vi "WS1050 Bench CAP Characterization_Ver1.2.vi"() -> ()   [LabVIEW 2012]
panel:
  in  "Tab Control":enum32{"CONTROL", "INDICATION"}(tab)
  in  "RFFE Com Port":refnum<visa-resource-name>="COM3"
  in  "AD7747 Com Port":refnum<visa-resource-name>="COM1"
  in  "Init":bool=TRUE
  in  "Wafer":string="WS1050"
  in  "Lot":string="Toggle 7"
  in  "SN":string="01"
  in  "Temperature":string="RT"
  in  "Delay(ms)":u32=100
  in  "TMN DC\\CAP Data Log File Path":path=path "C:/Andy Tr/Temp"
  in  "String":string="WS1050 BENCH CAP CHARACTERIZATION Ver1.2"
  out "C3Cal (pF)":dbl=-4.9974111328125
  out "C1Cal (pF)":dbl=-4.5642919921875
  out "C2Cal (pF)":dbl=-4.9191376953125
  out "S_ValueC3(pF)":dbl=-4.9974111328125
  out "S_ValueC1(pF)":dbl=-4.5642919921875
  out "S_ValueC2(pF)":dbl=-4.9191376953125
  in  "Calib Socket":bool
  out "C1_Mesa(pF)":dbl
  out "C2_Mesa(pF)":dbl
  out "C3_Mesa(pF)":dbl
  in  "A364X_VDD":refnum<visa-resource-name>="GPIB1::6::INSTR"
  in  "IDD Limit":dbl=0.02 format="%.2p"
  in  "VDD":dbl=3.3
  in  "CP Setting":i32(ring) items=["CP OFF", "CP ON", "DVA OFF", "DVA ON", "ECAL OFF", "ECAL ON", "CP 40.25V", "CP 35V", "CP 38V", "CP 44V", "CP 50V", "CP 23.75V", "CP 25.25V", "CP 29.75V", "C1 ON", "C1 OFF", "C2 ON", "C2 OFF", "C3 ON", "C3 OFF"]
  in  "Send":bool
  in  "Init AD7747":bool
  in  "Keithley 2000":refnum<visa-resource-name>
  in  "CApDac_values":string[](array[string])=["900b99", "900b99", "900b9b"]
  in  "Toggle Relay":bool
  in  "A3631E":refnum<visa-resource-name>
  in  "Channel":i32(ring)=1 items=["Channel 1"=1, "Channel 2"=2, "Channel 3"=3]
  in  "Relay Delay (s)":u32
  out "C_min(pF)":string[](array[string])
  out "C_Max":string[](array[string])
  out "C_Min2(pF)":string[](array[string])
  out "error out":errorcluster
  in  "error in (no error)":errorcluster
  in  "stop":bool
  in  "Abort":bool
  in  "Start Test":bool
  out "Running loop":i32
  in  "Set Cmax":string[](array[string])=["07413B", "07423B", "07433B"]
  out "Status":string="Relays Open..."
  # "This Version is working with V1.9 Marketing Firmware"
  # "Company:  WiSpry Inc\n198 Fairbanks Ste 198 Irvine\n\nCreated by:  Andy V Tran\nDate:  03/11/2015\nTP:  WS1050 Bench\nCAP Characterization"
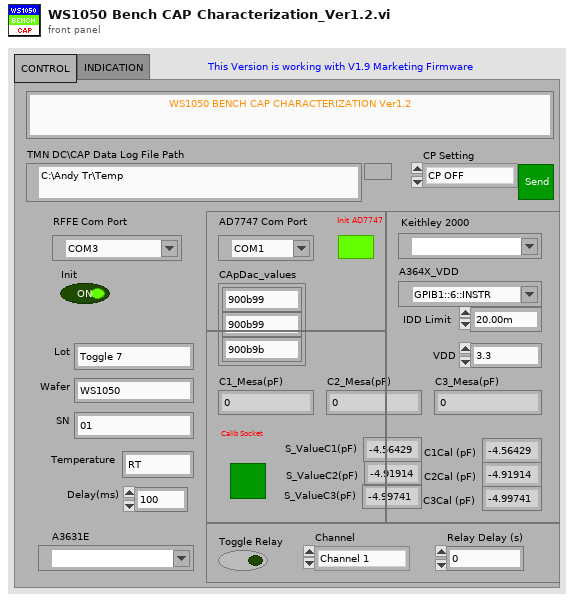
[diagram p1: front panel]
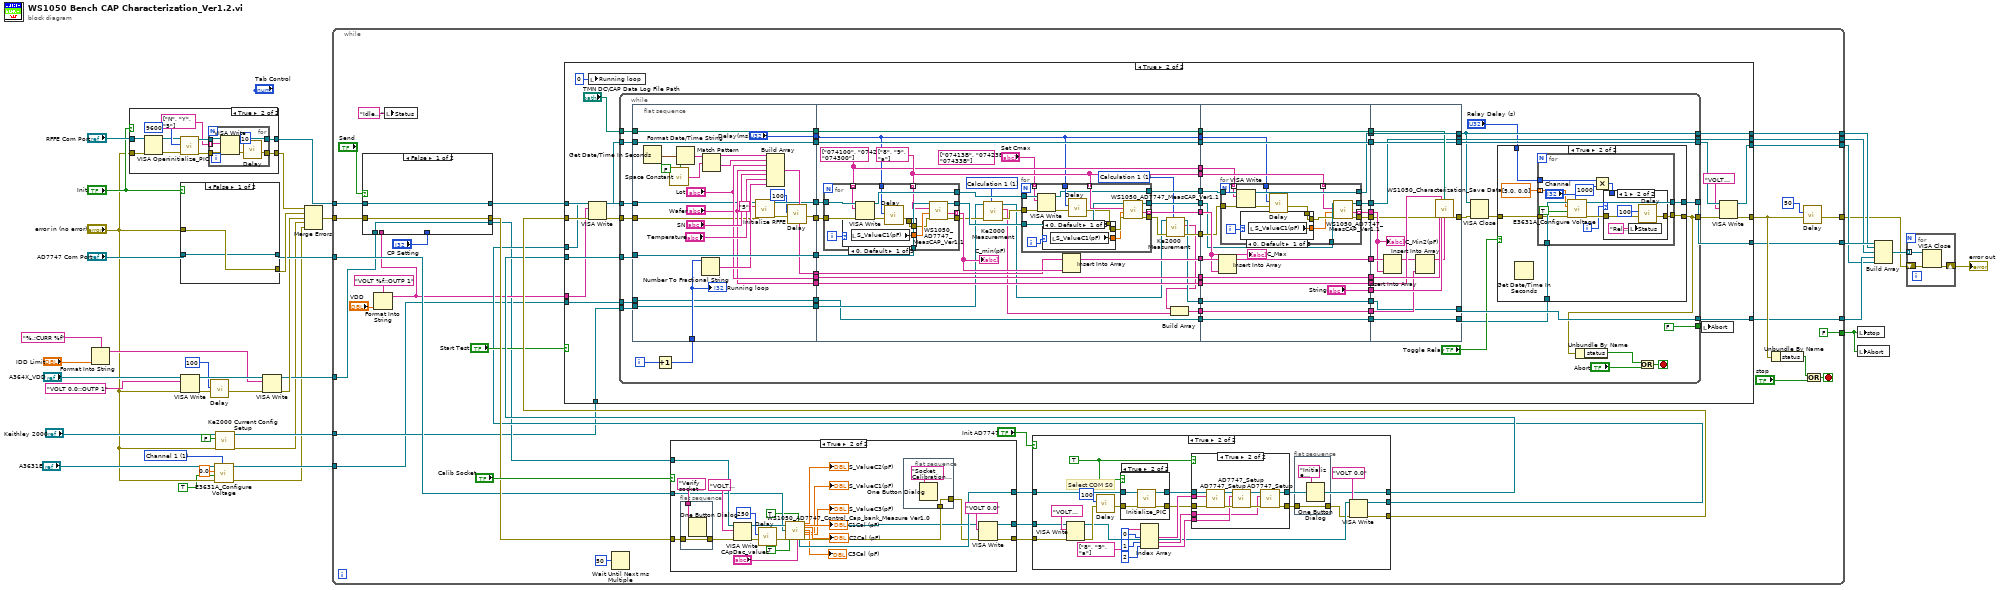
[diagram p0: block diagram]
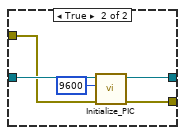
[diagram p3: hidden frame]
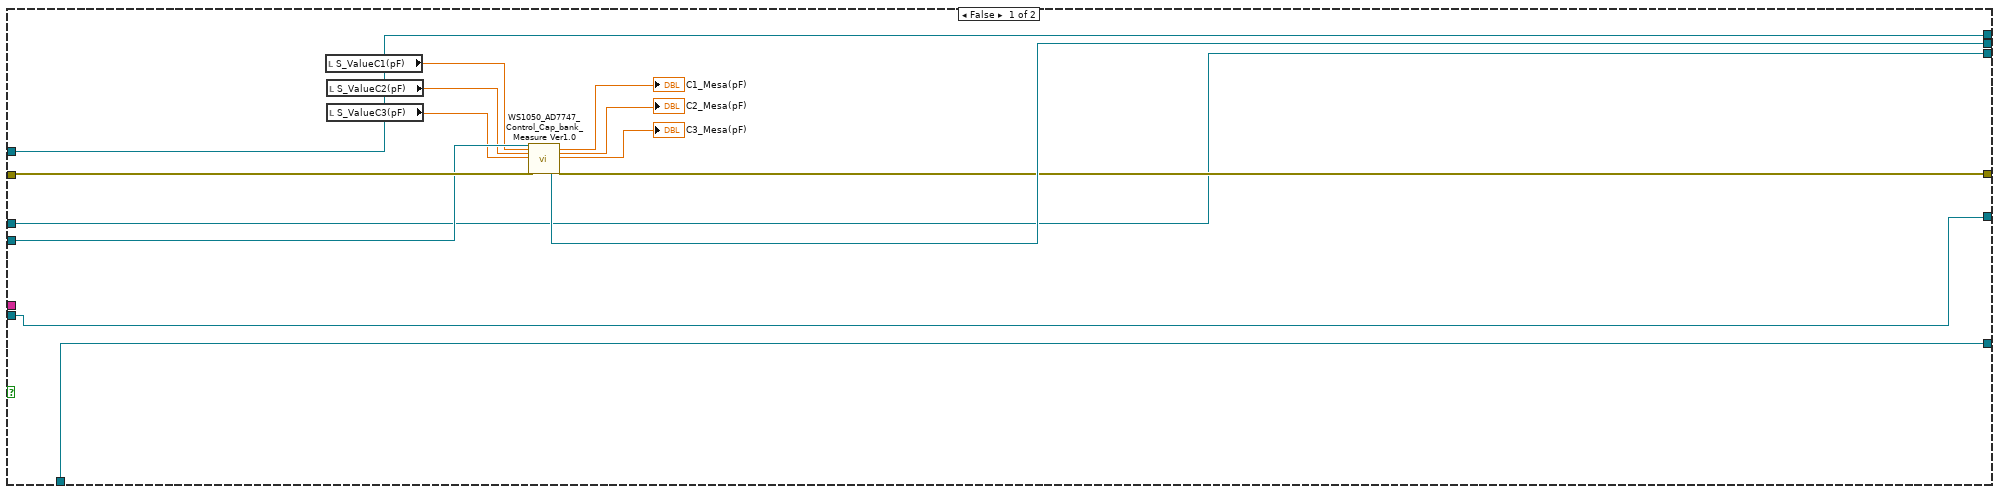
[diagram p8: hidden frame]
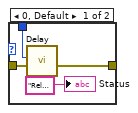
[diagram p10: hidden frame]
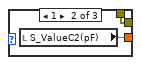
[diagram p11: hidden frame]
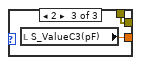
[diagram p12: hidden frame]
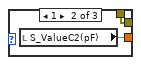
[diagram p13: hidden frame]
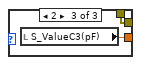
[diagram p14: hidden frame]
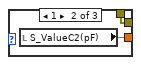
[diagram p15: hidden frame]
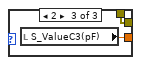
[diagram p16: hidden frame]
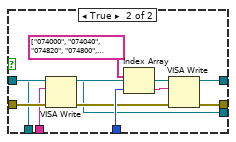
[diagram p17: hidden frame]
diagram:
  w13 = 1 items=["Channel 1"=1, "Channel 2"=2, "Channel 3"=3] ("Channel (1: Channel 1)")
  n1 = Format Into String(format string="%.;CURR %f", "IDD Limit") -> (resulting string=w34:string)  [unwired: 2 in, 1 out]
  n2 = case shown="True" "Init" {
    tunnel: "error in (no error)" -> [w41 w46]
    tunnel: [w41 w51] -> w17
    tunnel: "RFFE Com Port" -> [w40 w43]
    tunnel: [w40 w50] -> w18
    frame False {
    }
    frame True {
      n3 = VISA Open(error in (no error)=w46, VISA resource name=w43) -> (VISA resource name=w44:refnum<visa-resource-name>, error out=w45:errorcluster)  [unwired: 3 in]
      n4 = call "initialize_PIC.vi"("error in (no error)"=w45, "baud rate"=u32 9600, "Select Com Port"=w44) -> ("error out"=w48:errorcluster, "VISA resource name out"=w49:refnum<visa-resource-name>)  [unwired: 7 in]
      n5 = for {
        tunnel: [w58] -> w51
        tunnel: [w52] -> w50
        tunnel: w49 -> [w53]
        tunnel: w48 -> [w55]
        tunnel: string[] ["N", "Y", "5"] -> [w54] mode=indexing
        n6 = VISA Write(VISA resource name=w53, write buffer=w54, error in (no error)=w55) -> (VISA resource name out=w52:refnum<visa-resource-name>, error out=w56:errorcluster)  [unwired: 1 out]
        n7 = call "Delay.vi"("error in (no error)"=w56, "milliseconds to wait"=u32 10) -> ("error out"=w58:errorcluster)  [unwired: 9 in]
      }
    }
  }
  n8 = case shown="False" "Init" {
    tunnel: "AD7747 Com Port" -> [w59 w64]
    tunnel: [w60 w63] -> w38
    tunnel: [w59 w62] -> w37
    tunnel: "error in (no error)" -> [w60 w61]
    frame False {
    }
    frame True {
      n9 = call "Initialize_PIC.vi"("error in (no error)"=w61, "baud rate"=u32 9600, "Select Com Port"=w64) -> ("error out"=w63:errorcluster, "VISA resource name out"=w62:refnum<visa-resource-name>)  [unwired: 7 in]
    }
  }
  n10 = VISA Write(VISA resource name="A364X_VDD", write buffer="VOLT 0.0;:OUTP 1", error in (no error)="error in (no error)") -> (VISA resource name out=w35:refnum<visa-resource-name>, error out=w31:errorcluster)  [unwired: 1 out]
  n11 = call "Delay.vi"("error in (no error)"=w31, "milliseconds to wait"=u32 100) -> ("error out"=w36:errorcluster)  [unwired: 9 in]
  n12 = call "E3631A_Configure Voltage.vi"("Channel (1: Channel 1)"=w13, "error in (no error)"="error in (no error)", "Enable Output (T: Enable)"=TRUE, "Voltage(V)"=0.0, "VISA resource name"="A3631E") -> ("error out"=w10:errorcluster, "VISA resource name 2"=w11:refnum<visa-resource-name>)  [unwired: 5 in]
  n13 = call "Ke2000 Current Config Setup.vi"("error in (no error)"="error in (no error)", "Auto Range(T/F)"=FALSE, "VISA resource name"="Keithley 2000") -> ("error out"=w21:errorcluster, "VISA resource name out"=w22:refnum<visa-resource-name>)  [unwired: 7 in]
  n14 = VISA Write(VISA resource name=w35, write buffer=w34, error in (no error)=w36) -> (VISA resource name out=w26:refnum<visa-resource-name>, error out=w27:errorcluster)  [unwired: 1 out]
  n15 = Merge Errors(w17, w38, w27, w21, w10) -> (w9:errorcluster)
  n16 = while {
    tunnel: w18 -> [w99]
    tunnel: w9 -> [w100]
    tunnel: w37 -> [w87]
    tunnel: [w95] -> w2
    tunnel: [w93] -> w7
    tunnel: [w92] -> w6
    tunnel: w26 -> [w74]
    tunnel: [w78] -> w4
    tunnel: [FALSE ("stop")] -> w25
    tunnel: w22 -> [w70]
    tunnel: [w69] -> w5
    tunnel: w11 -> [w68]
    tunnel: [w67] -> w8
    stop <- w90 stop-if-true
    n17 = Format Into String(format string="VOLT %f;:OUTP 1", "VDD") -> (resulting string=w73:string)  [unwired: 2 in, 1 out]
    n18 = case shown="False" "Send" {
      tunnel: w100 -> [w469 w475]
      tunnel: [w469 w479] -> w88
      tunnel: [w468 w478] -> w98
      tunnel: "CP Setting" -> [_ w477]
      tunnel: w99 -> [w468 w476]
      tunnel: w74 -> [w467 w474]
      tunnel: w73 -> [_ w473]
      tunnel: [w467 w471] -> w72
      frame False {
      }
      frame True {
        n19 = VISA Write(VISA resource name=w474, write buffer=w473, error in (no error)=w475) -> (VISA resource name out=w471:refnum<visa-resource-name>, error out=w472:errorcluster)  [unwired: 1 out]
        n20 = Index Array(array=string[] ["074000", "074040", "074820", "074800", "074044", "074040", "074776", "07476F", "074773", "07477B", "07477C", "074760", "074762", "074768", "07413B", "074100", "07423B", "074200", "07433B", "074300"], index=w477) -> (element=w480:string)
        n21 = VISA Write(VISA resource name=w476, write buffer=w480, error in (no error)=w472) -> (VISA resource name out=w478:refnum<visa-resource-name>, error out=w479:errorcluster)  [unwired: 1 out]
      }
    }
    n22 = local write "Status"("Idle..." ("Status")) -> ()
    n23 = Wait Until Next ms Multiple(millisecond multiple=u32 50) -> ()  [unwired: 1 out]
    n24 = case shown="True" "Calib Socket" {
      tunnel: w88 -> [w153 w177]
      tunnel: [w153 w160] -> w82
      tunnel: w87 -> [w152 w158]
      tunnel: w72 -> [w151 w166]
      tunnel: [w151 w161] -> w83
      tunnel: [w152 w175] -> w81
      frame False {
      }
      frame True {
        n25 = flat-sequence {
          tunnel: [w180] -> w167
          tunnel: w177 -> [w180]
          tunnel: "Verify socket should be empty" ("message") -> [w179]
          frame #0 {
            n26 = One Button Dialog(message=w179) -> ()  [unwired: 1 in, 1 out]
          }
        }
        n27 = VISA Write(VISA resource name=w166, write buffer="VOLT 3.3;:OUTP 1", error in (no error)=w167) -> (VISA resource name out=w162:refnum<visa-resource-name>, error out=w164:errorcluster)  [unwired: 1 out]
        n28 = call "Delay.vi"("error in (no error)"=w164, "milliseconds to wait"=u32 250) -> ("error out"=w157:errorcluster)  [unwired: 9 in]
        n29 = call "WS1050_AD7747_Control_Cap_bank_Measure Ver1.0.vi"("Select Com Port"=w158, "errorin"=w157, "Push Button to Measue Cap"=TRUE, "CApDac_values"="CApDac_values", "Push Button to Calibrate"=TRUE ("Push Button to Initialize AD7747")) -> ("Com Port Out"=w175:refnum<visa-resource-name>, "C2(pF)"=→"S_ValueC2(pF)":dbl, "C1_Mesa(pF)"=→"C1Cal (pF)":dbl, "C2_Mesa(pF)"=→"C2Cal (pF)":dbl, "C3_Mesa(pF)"=→"C3Cal (pF)":dbl, "C1(pF)"=→"S_ValueC1(pF)":dbl, "C3(pF)"=→"S_ValueC3(pF)":dbl, "error out"=w176:errorcluster)  [unwired: 15 in]
        n30 = flat-sequence {
          tunnel: [w181] -> w159
          tunnel: w176 -> [w181]
          frame #0 {
            n31 = One Button Dialog(message="Socket Calibration Completed, Please insert DUT into the Socket") -> ()  [unwired: 1 in, 1 out]
          }
        }
        n32 = VISA Write(VISA resource name=w162, write buffer="VOLT 0.0", error in (no error)=w159) -> (VISA resource name out=w161:refnum<visa-resource-name>, error out=w160:errorcluster)  [unwired: 1 out]
      }
    }
    n33 = case shown="True" "Init AD7747" {
      tunnel: w81 -> [w104 w129]
      tunnel: [w105 w109] -> w85
      tunnel: w82 -> [w105 w114]
      tunnel: [w104 w107] -> w84
      tunnel: w83 -> [w103 w115]
      tunnel: [w103 w110] -> w79
      frame False {
      }
      frame True {
        w119 = TRUE
        # "Select COM S0"
        n34 = VISA Write(VISA resource name=w115, write buffer="VOLT 3.3;:OUTP 1", error in (no error)=w114) -> (VISA resource name out=w111:refnum<visa-resource-name>, error out=w113:errorcluster)  [unwired: 1 out]
        n35 = call "Delay.vi"("error in (no error)"=w113, "milliseconds to wait"=u32 100) -> ("error out"=w117:errorcluster)  [unwired: 9 in]
        n36 = case shown="True" w119 {
          tunnel: [w143 w148] -> w120
          tunnel: [w144 w147] -> w128
          tunnel: w129 -> [w144 w146]
          tunnel: w117 -> [w143 w145]
          frame False {
          }
          frame True {
            n37 = call "Initialize_PIC.vi"("error in (no error)"=w145, "Select Com Port"=w146) -> ("error out"=w148:errorcluster, "VISA resource name out"=w147:refnum<visa-resource-name>)  [unwired: 8 in]
          }
        }
        n38 = Index Array(array=string[] ["8", "9", "a"], index #1=0 ("index"), index #2=1 ("index"), index #3=2 ("index")) -> (element #1=w123:string, element #2=w122:string, element #3=w121:string)
        n39 = case shown="True" w119 {
          tunnel: w120 -> [w131 w134]
          tunnel: [w131 w132] -> w106
          tunnel: w128 -> [w130 w142]
          tunnel: w123 -> [_ w137]
          tunnel: w121 -> [_ w136]
          tunnel: w122 -> [_ w135]
          tunnel: [w130 w133] -> w107
          frame False {
          }
          frame True {
            n40 = call "AD7747_Setup.vi"("error in"=w134, "AD7747_Number"=w137, "Control"=w142) -> ("error out"=w141:errorcluster, "Control out"=w140:refnum<visa-resource-name>)  [unwired: 6 in, 1 out]
            n41 = call "AD7747_Setup.vi"("error in"=w141, "AD7747_Number"=w136, "Control"=w140) -> ("error out"=w139:errorcluster, "Control out"=w138:refnum<visa-resource-name>)  [unwired: 6 in, 1 out]
            n42 = call "AD7747_Setup.vi"("error in"=w139, "AD7747_Number"=w135, "Control"=w138) -> ("error out"=w132:errorcluster, "Control out"=w133:refnum<visa-resource-name>)  [unwired: 6 in, 1 out]
          }
        }
        n43 = flat-sequence {
          tunnel: w106 -> [w149]
          tunnel: [w149] -> w108
          frame #0 {
            n44 = One Button Dialog(message="Initialize AD7747 completed!") -> ()  [unwired: 1 in, 1 out]
          }
        }
        n45 = VISA Write(VISA resource name=w111, write buffer="VOLT 0.0", error in (no error)=w108) -> (VISA resource name out=w110:refnum<visa-resource-name>, error out=w109:errorcluster)  [unwired: 1 out]
      }
    }
    n46 = case shown="True" "Start Test" {
      tunnel: w98 -> [w189 w217]
      tunnel: w85 -> [w196 w212]
      tunnel: w84 -> [w195 w216]
      tunnel: [w193 w210] -> w96
      tunnel: [w189 w215] -> w93
      tunnel: [w194 w214] -> w92
      tunnel: w79 -> [w188 w211]
      tunnel: [w188 w207] -> w78
      tunnel: w73 -> [_ w202]
      tunnel: w70 -> [w184 w200]
      tunnel: [w184 w199] -> w69
      tunnel: w68 -> [w183 w198]
      tunnel: [w183 w197] -> w67
      frame False {
        n47 = local read "S_ValueC1(pF)"() -> (w187:dbl)
        n48 = local read "S_ValueC2(pF)"() -> (w186:dbl)
        n49 = local read "S_ValueC3(pF)"() -> (w185:dbl)
        n50 = call "WS1050_AD7747_Control_Cap_bank_Measure Ver1.0.vi"("Select Com Port"=w195, "S_Value C1"=w187, "S_Value C2"=w186, "S_Value C3"=w185, "errorin"=w196) -> ("Com Port Out"=w194:refnum<visa-resource-name>, "C1_Mesa(pF)"=→"C1_Mesa(pF)":dbl, "C2_Mesa(pF)"=→"C2_Mesa(pF)":dbl, "C3_Mesa(pF)"=→"C3_Mesa(pF)":dbl, "error out"=w193:errorcluster)  [unwired: 15 in, 3 out]
      }
      frame True {
        n51 = VISA Write(VISA resource name=w211, write buffer=w202, error in (no error)=w212) -> (VISA resource name out=w209:refnum<visa-resource-name>, error out=w213:errorcluster)  [unwired: 1 out]
        n52 = local write "Running loop"(0 ("Loop Running")) -> ()
        n53 = while {
          tunnel: w217 -> [w277]
          tunnel: w213 -> [w276]
          tunnel: w216 -> [w275]
          tunnel: [w218] -> w206
          tunnel: "TMN DC\\CAP Data Log File Path" -> [w270]
          tunnel: [w236] -> w215
          tunnel: [w266] -> w214
          tunnel: w209 -> [w262]
          tunnel: [w259] -> w208
          tunnel: [FALSE ("Abort")] -> w203
          tunnel: w200 -> [w234]
          tunnel: [w228] -> w199
          tunnel: w198 -> [w225]
          tunnel: [w220] -> w197
          i -> [w253]
          stop <- w272 stop-if-true
          n54 = flat-sequence {
            tunnel: w262 -> [w332]
            tunnel: w270 -> [w333]
            tunnel: w275 -> [w334]
            tunnel: w276 -> [w315]
            tunnel: w277 -> [w316]
            tunnel: [w312] -> w251
            tunnel: [w313] -> w250
            tunnel: [w334] -> w249
            tunnel: [w333] -> w248
            tunnel: [w332] -> w247
            tunnel: w246 -> [w319]
            tunnel: [w322] -> w245
            tunnel: ["Lot"] -> w244
            tunnel: ["Wafer"] -> w241
            tunnel: ["Delay(ms)"] -> w237
            tunnel: w234 -> [w310]
            tunnel: [w310] -> w233
            tunnel: w225 -> [w309]
            tunnel: [w309] -> w224
            tunnel: [w356] -> w280
            tunnel: [w361] -> w279
            tunnel: [w343] -> w274
            tunnel: [w360] -> w269
            tunnel: [w359] -> w267
            tunnel: [w358] -> w264
            tunnel: [w355] -> w260
            tunnel: [w354] -> w258
            tunnel: [w349] -> w257
            tunnel: [w353] -> w256
            tunnel: w251 -> [w366]
            tunnel: w250 -> [w365]
            tunnel: w249 -> [w363]
            tunnel: w248 -> [w358]
            tunnel: w247 -> [w355]
            tunnel: w245 -> [w352]
            tunnel: w244 -> [w351]
            tunnel: [w351] -> w243
            tunnel: w241 -> [w350]
            tunnel: [w350] -> w240
            tunnel: w237 -> [w349]
            tunnel: w233 -> [w346]
            tunnel: [w341] -> w232
            tunnel: [w337] -> w230
            tunnel: w224 -> [w335]
            tunnel: [w335] -> w223
            tunnel: w280 -> [w429]
            tunnel: w279 -> [w428]
            tunnel: [w427] -> w278
            tunnel: w274 -> [w423]
            tunnel: [w424] -> w273
            tunnel: w269 -> [w419]
            tunnel: [w418] -> w268
            tunnel: w267 -> [w417]
            tunnel: [w426] -> w265
            tunnel: w264 -> [w426]
            tunnel: [w425] -> w261
            tunnel: w260 -> [w425]
            tunnel: w258 -> [w422]
            tunnel: w257 -> [w421]
            tunnel: w256 -> [w420]
            tunnel: [w416] -> w255
            tunnel: [w415] -> w254
            tunnel: w243 -> [w414]
            tunnel: [w414] -> w242
            tunnel: w240 -> [w413]
            tunnel: [w413] -> w239
            tunnel: ["String"] -> w238
            tunnel: w232 -> [w411]
            tunnel: [w411] -> w231
            tunnel: w230 -> [w410]
            tunnel: [w410] -> w229
            tunnel: w223 -> [w409]
            tunnel: [w409] -> w222
            tunnel: w278 -> [w461]
            tunnel: w273 -> [w456]
            tunnel: [w466] -> w235
            tunnel: w268 -> [w465]
            tunnel: [w465] -> w236
            tunnel: [w462] -> w266
            tunnel: w265 -> [w464]
            tunnel: w261 -> [w463]
            tunnel: [w463] -> w259
            tunnel: w255 -> [w462]
            tunnel: w254 -> [w460]
            tunnel: w242 -> [w459]
            tunnel: w239 -> [w458]
            tunnel: w238 -> [w457]
            tunnel: w231 -> [w452]
            tunnel: w229 -> [w454]
            tunnel: [w452] -> w228
            tunnel: w222 -> [w451]
            tunnel: [w451] -> w221
            frame #0 {
              n55 = Get Date/Time In Seconds() -> (seconds since 1Jan1904=w328:timestamp)
              n56 = call <vilib>:"Space Constant.vi"() -> ("String"=w331:string)
              n57 = Format Date/Time String(seconds (now)=w328, UTC format=FALSE) -> (date/time string=w329:string)  [unwired: 1 out]
              n58 = Number To Fractional String(number=w319) -> (F-format string=w323:string)  [unwired: 3 in]
              n59 = Match Pattern(string=w329, regular expression=w331) -> (before substring=w327:string, after substring=w326:string)  [unwired: 3 out]
              n60 = call "Initialize RFFE.vi"("error in (no error)"=w315, "write buffer"="5", "Select Com Port"=w316) -> ("error out"=w314:errorcluster, "VISA resource name out"=w312:refnum<visa-resource-name>)  [unwired: 7 in]
              n61 = Build Array(w327, w326, "Lot", "Wafer", "SN", "Temperature", w323) -> (w322:string[])
              n62 = call "Delay.vi"("error in (no error)"=w314, "milliseconds to wait"=u32 100) -> ("error out"=w313:errorcluster)  [unwired: 9 in]
              "Running loop" <- w319
            }
            frame #1 {
              w340 = u16 1 items=["Function", "Calculation 1", "Calculation 2", "Calculation 3"] ("Source (0: Function)")
              w345 = u16 1 items=["Function", "Calculation 1", "Calculation 2", "Calculation 3"] ("Source (0: Function)")
              w354 = string[] ["8", "9", "a"]
              (unwired) string[] ["07413B", "07423B", "07433B"]
              w353 = string[] ["074100", "074200", "074300"]
              n63 = for {
                tunnel: w366 -> [w402]
                tunnel: w365 -> [w401]
                tunnel: w353 -> [w400] mode=indexing
                tunnel: [w399] -> w364
                tunnel: w363 -> [w398]
                tunnel: [w397] -> w362
                tunnel: [w396] -> w347
                tunnel: w349 -> [w394]
                tunnel: w354 -> [w393] mode=indexing
                tunnel: [w392] -> w357 mode=indexing
                i -> [w391]
                n64 = VISA Write(VISA resource name=w402, write buffer=w400, error in (no error)=w401) -> (VISA resource name out=w399:refnum<visa-resource-name>, error out=w395:errorcluster)  [unwired: 1 out]
                n65 = call "Delay.vi"("error in (no error)"=w395, "milliseconds to wait"=w394) -> ("error out"=w389:errorcluster)  [unwired: 9 in]
                n66 = case shown="0, Default" w391 {
                  tunnel: [w404 w406 w408] -> w390
                  tunnel: w389 -> [w403 w405 w407]
                  tunnel: [w403 w405 w407] -> w388
                  frame 0, Default {
                    n67 = local read "S_ValueC1(pF)"() -> (w404:dbl)
                  }
                  frame 1 {
                    n68 = local read "S_ValueC2(pF)"() -> (w406:dbl)
                  }
                  frame 2 {
                    n69 = local read "S_ValueC3(pF)"() -> (w408:dbl)
                  }
                }
                n70 = call "WS1050_AD7747_MeasCAP_Ver1.1.vi"("error in (no error)"=w388, "OFFSet Cal"=w390, "AD7747_Number"=w393, "Control"=w398) -> ("error"=w396:errorcluster, "CAP (pF)"=w392:string, "Control out"=w397:refnum<visa-resource-name>)  [unwired: 3 in, 2 out]
              }
              "C_min(pF)" <- w357
              n71 = call "Ke2000 Measurement.vi"("Source (0: Function)"=w345, "error in (no error)"=w347, "VISA resource name"=w346) -> ("error out"=w348:errorcluster, "Meas in micro"=w338:string, "VISA resource name out"=w342:refnum<visa-resource-name>)  [unwired: 3 in, 3 out]
              n72 = for {
                tunnel: w364 -> [w381]
                tunnel: w348 -> [w380]
                tunnel: "Set Cmax" -> [w379] mode=indexing
                tunnel: w349 -> [w377]
                tunnel: w354 -> [w376] mode=indexing
                tunnel: [w375] -> w344
                tunnel: [w374] -> w359
                tunnel: [w373] -> w360
                tunnel: w362 -> [w372]
                tunnel: [w371] -> w361 mode=indexing
                i -> [w369]
                n73 = VISA Write(VISA resource name=w381, write buffer=w379, error in (no error)=w380) -> (VISA resource name out=w373:refnum<visa-resource-name>, error out=w378:errorcluster)  [unwired: 1 out]
                n74 = call "Delay.vi"("error in (no error)"=w378, "milliseconds to wait"=w377) -> ("error out"=w368:errorcluster)  [unwired: 9 in]
                n75 = case shown="0, Default" w369 {
                  tunnel: [w383 w385 w387] -> w367
                  tunnel: w368 -> [w382 w384 w386]
                  tunnel: [w382 w384 w386] -> w370
                  frame 0, Default {
                    n76 = local read "S_ValueC1(pF)"() -> (w383:dbl)
                  }
                  frame 1 {
                    n77 = local read "S_ValueC2(pF)"() -> (w385:dbl)
                  }
                  frame 2 {
                    n78 = local read "S_ValueC3(pF)"() -> (w387:dbl)
                  }
                }
                n79 = call "WS1050_AD7747_MeasCAP_Ver1.1.vi"("error in (no error)"=w370, "OFFSet Cal"=w367, "AD7747_Number"=w376, "Control"=w372) -> ("error"=w375:errorcluster, "CAP (pF)"=w371:string, "Control out"=w374:refnum<visa-resource-name>)  [unwired: 3 in, 2 out]
              }
              n80 = Insert Into Array(array=w352, new element=w357) -> (w356:string[])  [unwired: 1 in]
              n81 = call "Ke2000 Measurement.vi"("Source (0: Function)"=w340, "error in (no error)"=w344, "VISA resource name"=w342) -> ("error out"=w343:errorcluster, "Meas in micro"=w339:string, "VISA resource name out"=w341:refnum<visa-resource-name>)  [unwired: 3 in, 3 out]
              n82 = Build Array(w339, w338) -> (w337:string[])
            }
            frame #2 {
              n83 = Insert Into Array(array=w429, new element=w428) -> (w427:string[])  [unwired: 1 in]
              n84 = for {
                tunnel: w419 -> [w444]
                tunnel: w423 -> [w443]
                tunnel: w420 -> [w442] mode=indexing
                tunnel: [w441] -> w418
                tunnel: w417 -> [w440]
                tunnel: [w439] -> w416
                tunnel: [w438] -> w424
                tunnel: w421 -> [w436]
                tunnel: w422 -> [w435] mode=indexing
                tunnel: [w434] -> w415 mode=indexing
                i -> [w433]
                n85 = VISA Write(VISA resource name=w444, write buffer=w442, error in (no error)=w443) -> (VISA resource name out=w441:refnum<visa-resource-name>, error out=w437:errorcluster)  [unwired: 1 out]
                n86 = call "Delay.vi"("error in (no error)"=w437, "milliseconds to wait"=w436) -> ("error out"=w431:errorcluster)  [unwired: 9 in]
                n87 = case shown="0, Default" w433 {
                  tunnel: [w446 w448 w450] -> w430
                  tunnel: w431 -> [w445 w447 w449]
                  tunnel: [w445 w447 w449] -> w432
                  frame 0, Default {
                    n88 = local read "S_ValueC1(pF)"() -> (w446:dbl)
                  }
                  frame 1 {
                    n89 = local read "S_ValueC2(pF)"() -> (w448:dbl)
                  }
                  frame 2 {
                    n90 = local read "S_ValueC3(pF)"() -> (w450:dbl)
                  }
                }
                n91 = call "WS1050_AD7747_MeasCAP_Ver1.1.vi"("error in (no error)"=w432, "OFFSet Cal"=w430, "AD7747_Number"=w435, "Control"=w440) -> ("error"=w438:errorcluster, "CAP (pF)"=w434:string, "Control out"=w439:refnum<visa-resource-name>)  [unwired: 3 in, 2 out]
              }
              "C_Max" <- w428
            }
            frame #3 {
              n92 = Insert Into Array(array=w461, new element=w460) -> (w455:string[])  [unwired: 1 in]
              n93 = Insert Into Array(array=w455, new element=w454) -> (w453:string[])  [unwired: 1 in]
              n94 = call "WS1050_Characterization_Save Data.vi"("error in (no error)"=w456, "Lot"=w459, "Wafer"=w458, "TP"=w457, "TMN DC\\CAP Data Log File Path"=w464, "All Out"=w453) -> ("error out"=w466:errorcluster)  [unwired: 19 in, 2 out]
              "C_Min2(pF)" <- w460
            }
          }
          n95 = Increment(x=w253) -> (x+1=w246:i32)
          n96 = VISA Close(VISA resource name=w236, error in (no error)=w235) -> (error out=w227:errorcluster)
          n97 = case shown="True" "Toggle Relay" {
            tunnel: w227 -> [w282 w288]
            tunnel: [w282 w287] -> w218
            tunnel: w221 -> [w281 w286]
            tunnel: [w281 w285] -> w220
            tunnel: "Relay Delay (s)" -> [_ w283]
            frame False {
            }
            frame True {
              n98 = Get Date/Time In Seconds() -> ()  [unwired: 1 out]
              n99 = for {
                tunnel: w288 -> [w297]
                tunnel: [w300] -> w287
                tunnel: w286 -> [w298]
                tunnel: [w295] -> w285
                tunnel: dbl[] [5.0, 0.0] -> [w293] mode=indexing
                tunnel: w283 -> [w292]
                i -> [w289]
                n100 = call "E3631A_Configure Voltage.vi"("Channel (1: Channel 1)"="Channel", "error in (no error)"=w297, "Enable Output (T: Enable)"=TRUE, "Voltage(V)"=w293, "VISA resource name"=w298) -> ("error out"=w299:errorcluster, "VISA resource name 2"=w295:refnum<visa-resource-name>)  [unwired: 5 in]
                n101 = Multiply(x=w292, y=u32 1000) -> (x*y=w290:u32)
                n102 = case shown="1" w289 {
                  tunnel: [w304 w308] -> w300
                  tunnel: w299 -> [w303 w307]
                  tunnel: w290 -> [w302 _]
                  frame 0, Default {
                    n103 = call "Delay.vi"("error in (no error)"=w303, "milliseconds to wait"=w302) -> ("error out"=w304:errorcluster)  [unwired: 9 in]
                    "Status" <- "Relays Open! Waiting for the next measurement..."
                  }
                  frame 1 {
                    n104 = local write "Status"("Relays Close! Measuring..." ("Status")) -> ()
                    n105 = call "Delay.vi"("error in (no error)"=w307, "milliseconds to wait"=u32 100) -> ("error out"=w308:errorcluster)  [unwired: 9 in]
                  }
                }
              }
            }
          }
          n106 = Unbundle By Name(w218) -> ("status"=w271:bool)
          n107 = Or(x=w271, y="Abort") -> (x .or. y?=w272:bool)
        }
        n108 = local write "Abort"(w203) -> ()
        n109 = VISA Write(VISA resource name=w208, write buffer="VOLT 0.0;:OUTP 0", error in (no error)=w206) -> (VISA resource name out=w207:refnum<visa-resource-name>, error out=w210:errorcluster)  [unwired: 1 out]
      }
    }
    n110 = Unbundle By Name(w96) -> ("status"=w97:bool)
    n111 = call "Delay.vi"("error in (no error)"=w96, "milliseconds to wait"=u32 50) -> ("error out"=w95:errorcluster)  [unwired: 9 in]
    n112 = Or(x=w97, y="stop") -> (x .or. y?=w90:bool)
  }
  n113 = local write "stop"(w25) -> ()
  n114 = local write "Abort"(w25) -> ()
  n115 = Build Array(w8, w7, w6, w5, w4) -> (w3:refnum<visa-resource-name>[])
  n116 = for {
    tunnel: w3 -> [w483] mode=indexing
    shift-right: [w481] -> w1
    shift-left: w2 -> [w482]
    n117 = VISA Close(VISA resource name=w483, error in (no error)=w482) -> (error out=w481:errorcluster)
  }
  "error out" <- w1
